vi "put_tablecloth.vi"(8 "error in (no error)":errorcluster, 11 "ITable in":refnum<class "ITable.lvclass">) -> (0 "error out":errorcluster, 2 "result":string, 3 "ITable out":refnum<class "ITable.lvclass">)   [LabVIEW 2021, in "ITable.lvclass"]
uses:
  ITable.lvclass
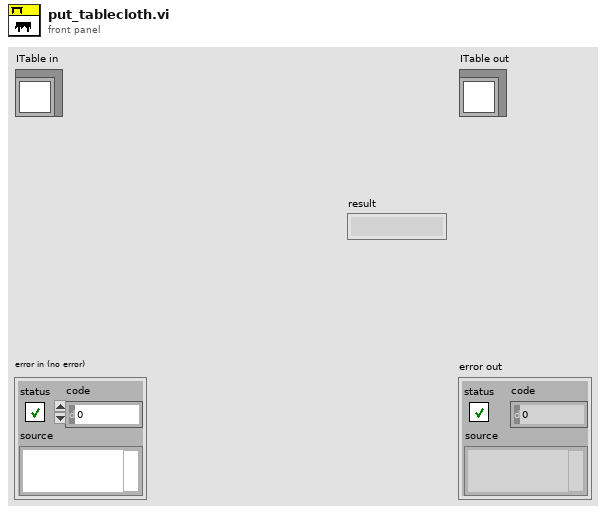
[diagram p1: front panel]
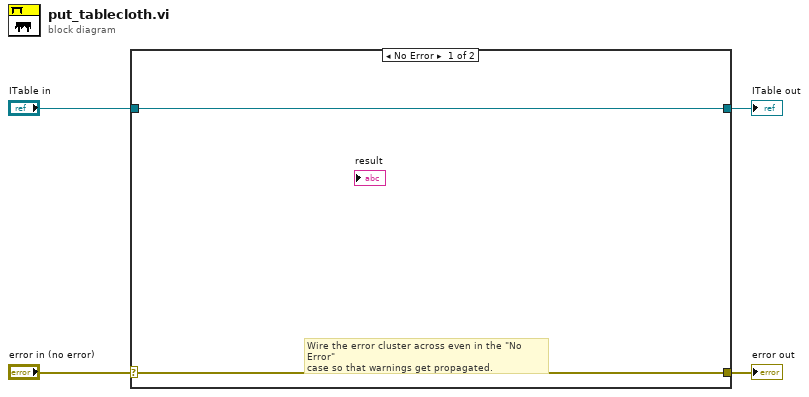
[diagram p0: block diagram]
diagram:
  n1 = case shown="No Error" "error in (no error)" {
    selector: "error in (no error)" -> [w5 w8]
    tunnel: [w5 w8] -> w3
    tunnel: [w6 w7] -> w1
    tunnel: "ITable in" -> [w6 w7]
    frame No Error {
      # "Wire the error cluster across even in the \"No Error\"\ncase so that warnings get propagated."
    }
    frame Error {
    }
  }
  "error out" <- w3
  "ITable out" <- w1
